vi "ramp_by_delta_double.vi"(9 "start":dbl format="%0.2f", 10 "end":dbl=1.0 format="%0.2f", 11 "delta":dbl=0.125) -> (3 "Ramp Pattern":dbl[](array[numeric]))   [LabVIEW 2019]
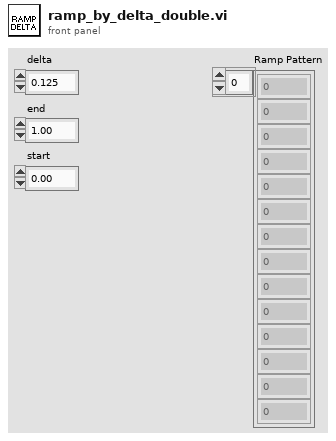
[diagram p1: front panel]
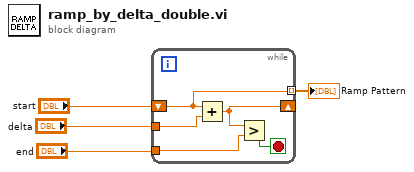
[diagram p0: block diagram]
diagram:
  n1 = while {
    shift-right: [w7] -> _
    shift-left: "start" -> [w5]
    tunnel: "delta" -> [w9]
    tunnel: "end" -> [w6]
    tunnel: [w5] -> w1 mode=indexing
    stop <- w8 stop-if-true
    n2 = Add(x=w5, y=w9) -> (x+y=w7:dbl)
    n3 = Greater?(x=w7, y=w6) -> (0:w8:bool)
  }
  "Ramp Pattern" <- w1
